vi "init.vi"(8 "error in (no error)":errorcluster, 11 "DualActingPneumaticCylinder in":refnum<class "DualActingPneumaticCylinder.lvclass">) -> (0 "error out":errorcluster, 3 "DualActingPneumaticCylinder out":refnum<class "DualActingPneumaticCylinder.lvclass">)   [LabVIEW 2013, in "DualActingPneumaticCylinder.lvclass"]
uses:
  DualActingPneumaticCylinder.lvclass
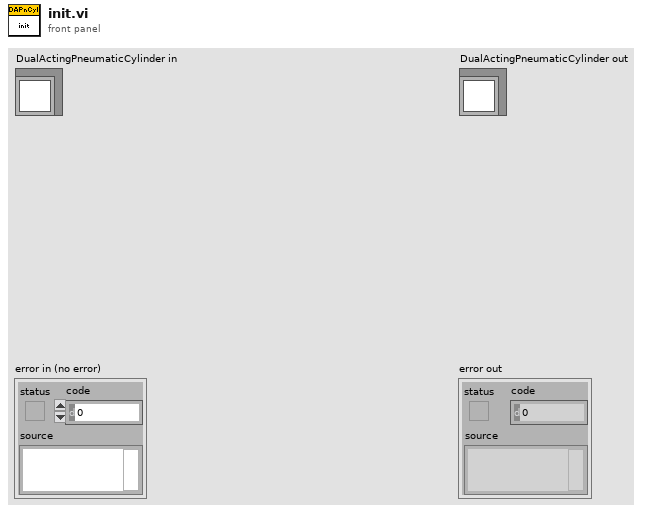
[diagram p1: front panel]
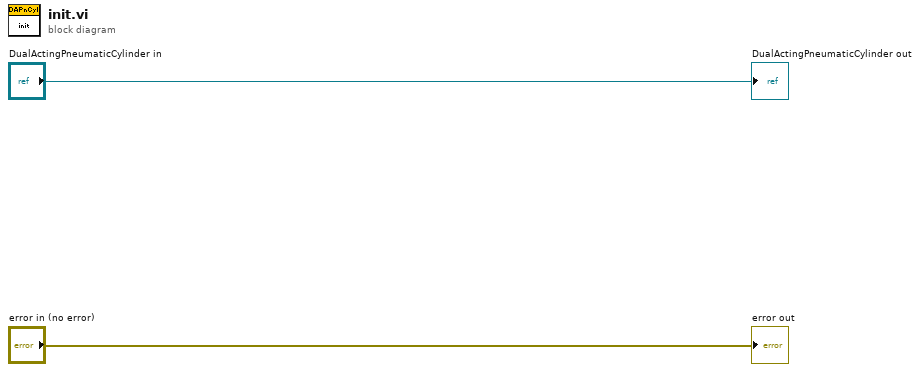
[diagram p0: block diagram]
diagram:
  "error out" <- "error in (no error)"
  "DualActingPneumaticCylinder out" <- "DualActingPneumaticCylinder in"
